vi "Application Note Input Data.vi"() -> ()   [LabVIEW 2020]
panel:
  out "웨이브폼 그래프":i8[](graph)
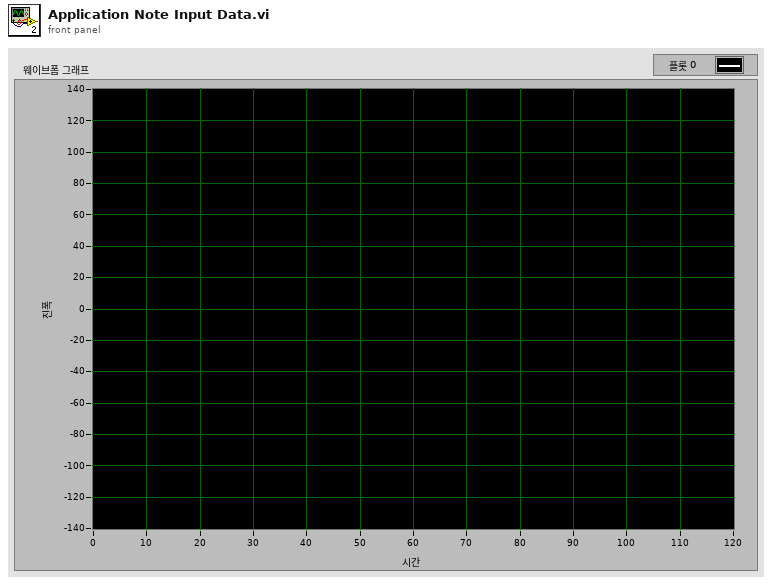
[diagram p1: front panel]
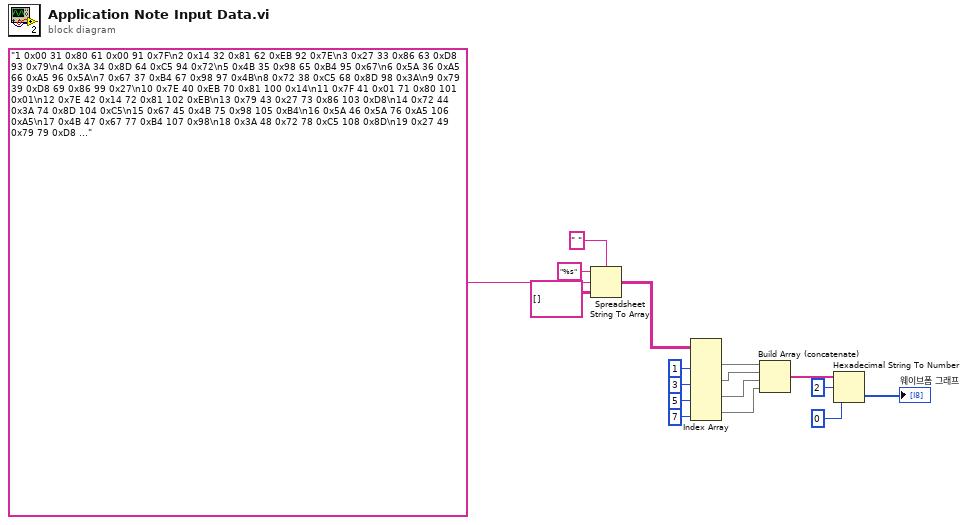
[diagram p0: block diagram]
diagram:
  n1 = Spreadsheet String To Array(delimiter (Tab)=" " ("구분 문자 (탭)"), format string="%s" ("포맷 문자열"), spreadsheet string="1 0x00 31 0x80 61 0x00 91 0x7F\n2 0x14 32 0x81 62 0xEB 92 0x7E\n3 0x27 33 0x86 63 0xD8 93 0x79\n4 0x3A 34 0x8D 64 0xC5 94 0x72\n5 0x4B 35 0x98 65 0xB4 95 0x67\n6 0x5A 36 0xA5 66 0xA5 96 0x5A\n7 0x67 37 0xB4 67 0x98 97 0x4B\n8 0x72 38 0xC5 68 0x8D 98 0x3A\n9 0x79 39 0xD8 69 0x86 99 0x27\n10 0x7E 40 0xEB 70 0x81 100 0x14\n11 0x7F 41 0x01 71 0x80 101 0x01\n12 0x7E 42 0x14 72 0x81 102 0xEB\n13 0x79 43 0x27 73 0x86 103 0xD8\n14 0x72 44 0x3A 74 0x8D 104 0xC5\n15 0x67 45 0x4B 75 0x98 105 0xB4\n16 0x5A 46 0x5A 76 0xA5 106 0xA5\n17 0x4B 47 0x67 77 0xB4 107 0x98\n18 0x3A 48 0x72 78 0xC5 108 0x8D\n19 0x27 49 0x79 79 0xD8 109 0x86\n20 0x14 50 0x7E 80 0xEB 110 0x81\n21 0x00 51 0x7F 81 0x01 111 0x80\n22 0xEB 52 0x7E 82 0x14 112 0x81\n23 0xD8 53 0x79 83 0x27 113 0x86\n24 0xC5 54 0x72 84 0x3A 114 0x8D\n25 0xB4 55 0x67 85 0x4B 115 0x98\n26 0xA5 56 0x5A 86 0x5A 116 0xA5\n27 0x98 57 0x4B 87 0x67 117 0xB4\n28 0x8D 58 0x3A 88 0x72 118 0xC5\n29 0x86 59 0x27 89 0x79 119 0xD8\n30 0x81 60 0x14 90 0x7E 120 0xEB", array type (2D Dbl)=string[][] [] ("배열 타입(2D Dbl)")) -> (array=w13:string[][])
  n2 = Index Array(array=w13, index (col) #1=1 ("비활성화된 인덱스 (열)"), index (col) #2=3 ("인덱스 (열)"), index (col) #3=5 ("인덱스 (열)"), index (col) #4=7 ("인덱스 (열)")) -> (element #1=w9:string[], element #2=w8:string[], element #3=w7:string[], element #4=w1:string[])  [unwired: 4 in]
  n3 = Build Array (concatenate)(w9, w8, w7, w1) -> (w6:string[])
  n4 = Hexadecimal String To Number(string=w6, offset=2 ("오프셋"), default (0uL)=i8 0 ("기본(0 U32)")) -> (number=→"웨이브폼 그래프":i8[])  [unwired: 1 out]
